vi "Add Item to Target.vi"(8 "error in (no error)":errorcluster, 10 "New Item Path":path, 11 "TargetRef In":refnum<vi>) -> (0 "error out":errorcluster, 3 "TargetRef Out":refnum<vi>)   [LabVIEW 2015, in "Generic Module Library.lvlib"]
uses:
  Generic Module Library.lvlib
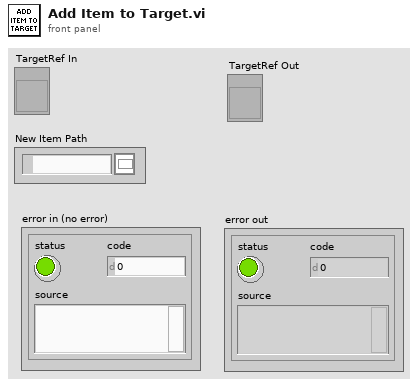
[diagram p1: front panel]
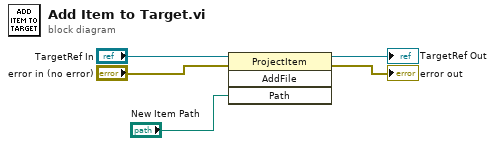
[diagram p0: block diagram]
diagram:
  n1 = invoke class="ProjectItem" method="AddFile"(reference="TargetRef In", error in="error in (no error)", "Path"="New Item Path") -> (reference out=→"TargetRef Out":refnum<vi>, error out=→"error out":errorcluster)  [unwired: 1 in, 2 out]
